vi "Set CCD_Config.vi"(8 "error in (no error)":errorcluster, 10 "input cluster":T1, 11 "Interface in":refnum<class "Interface.lvclass">) -> (0 "error out":errorcluster, 3 "Interface out":refnum<class "Interface.lvclass">)   [LabVIEW 2018, in "Interface.lvclass"]
uses:
  Interface.lvclass
  Interface.lvclass/Interface.ctl
panel:
  in  "EXPTIME":dbl
  in  "#FRAMES":u32
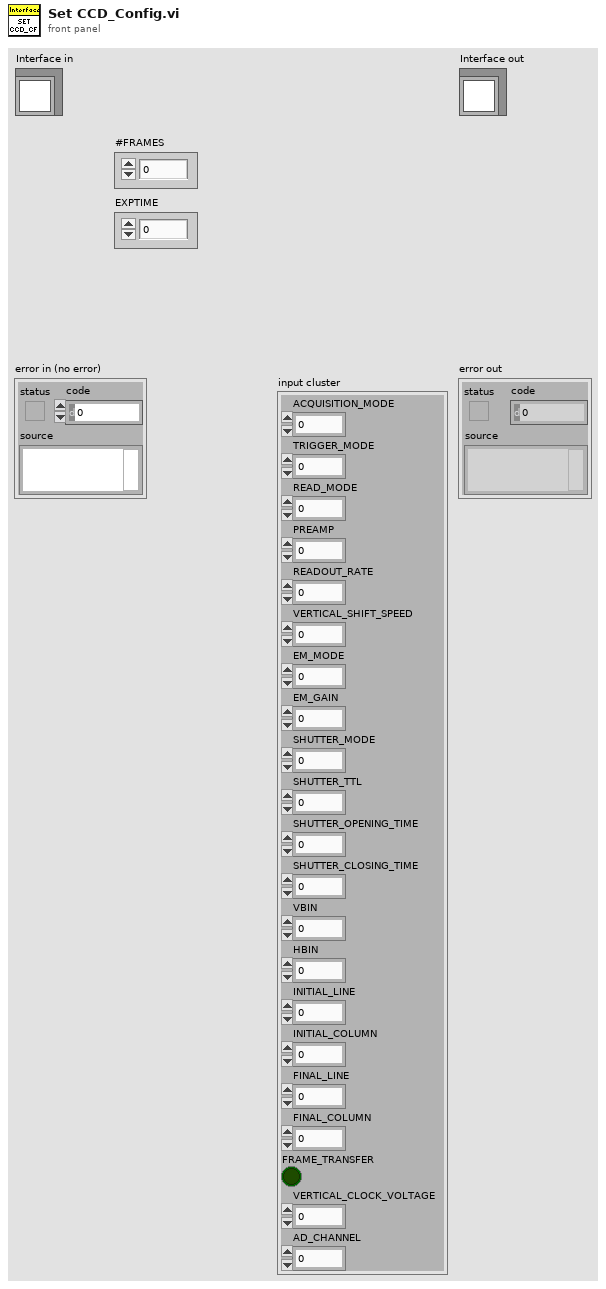
[diagram p1: front panel]
types:
  T1 = cluster{"ACQUISITION_MODE":u8, "TRIGGER_MODE":u8, "READ_MODE":u8, "PREAMP":u8, "READOUT_RATE":u8, "VERTICAL_SHIFT_SPEED":u8, "EM_MODE":u8, "EM_GAIN":u16, "SHUTTER_MODE":u8, "SHUTTER_TTL":u8, "SHUTTER_OPENING_TIME":u16, "SHUTTER_CLOSING_TIME":u16, "VBIN":u16, "HBIN":u16, "INITIAL_LINE":u16, "INITIAL_COLUMN":u16, "FINAL_LINE":u16, "FINAL_COLUMN":u16, "FRAME_TRANSFER":bool, "VERTICAL_CLOCK_VOLTAGE":u8, "AD_CHANNEL":u32}
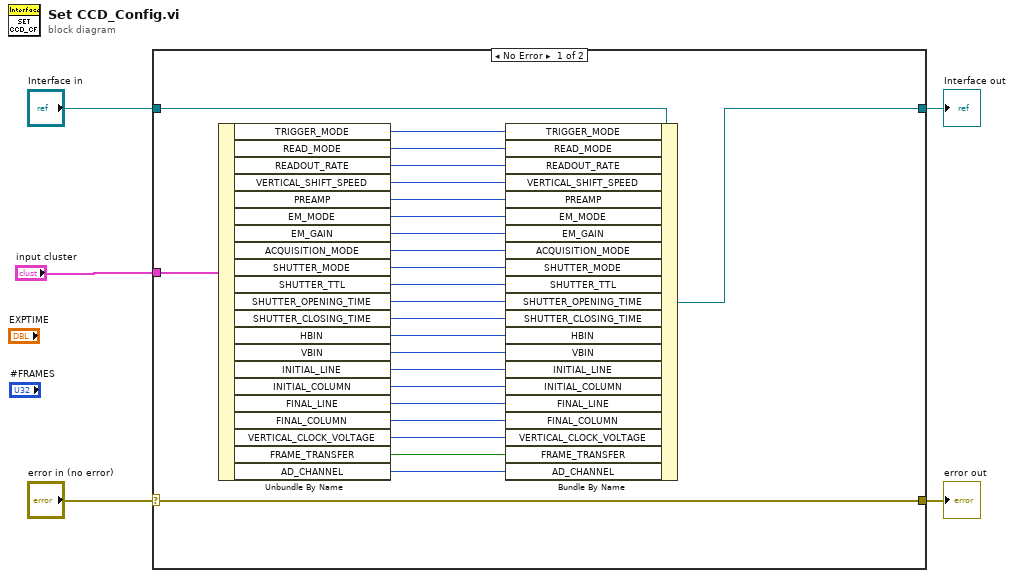
[diagram p0: block diagram]
diagram:
  n1 = case shown="No Error" "error in (no error)" {
    selector: "error in (no error)" -> [w30 w32]
    tunnel: [w30 w32] -> w4
    tunnel: [w6 w31] -> w2
    tunnel: "Interface in" -> [w7 w31]
    tunnel: "input cluster" -> [w8 _]
    frame No Error {
      n2 = Unbundle By Name(w8) -> ("TRIGGER_MODE"=w29:u8, "READ_MODE"=w28:u8, "READOUT_RATE"=w27:u8, "VERTICAL_SHIFT_SPEED"=w26:u8, "PREAMP"=w25:u8, "EM_MODE"=w24:u8, "EM_GAIN"=w23:u16, "ACQUISITION_MODE"=w22:u8, "SHUTTER_MODE"=w21:u8, "SHUTTER_TTL"=w20:u8, "SHUTTER_OPENING_TIME"=w19:u16, "SHUTTER_CLOSING_TIME"=w18:u16, "HBIN"=w17:u16, "VBIN"=w16:u16, "INITIAL_LINE"=w15:u16, "INITIAL_COLUMN"=w14:u16, "FINAL_LINE"=w13:u16, "FINAL_COLUMN"=w12:u16, "VERTICAL_CLOCK_VOLTAGE"=w11:u8, "FRAME_TRANSFER"=w10:bool, "AD_CHANNEL"=w9:u32)
      n3 = Bundle By Name(cluster=w7, "TRIGGER_MODE"=w29, "READ_MODE"=w28, "READOUT_RATE"=w27, "VERTICAL_SHIFT_SPEED"=w26, "PREAMP"=w25, "EM_MODE"=w24, "EM_GAIN"=w23, "ACQUISITION_MODE"=w22, "SHUTTER_MODE"=w21, "SHUTTER_TTL"=w20, "SHUTTER_OPENING_TIME"=w19, "SHUTTER_CLOSING_TIME"=w18, "HBIN"=w17, "VBIN"=w16, "INITIAL_LINE"=w15, "INITIAL_COLUMN"=w14, "FINAL_LINE"=w13, "FINAL_COLUMN"=w12, "VERTICAL_CLOCK_VOLTAGE"=w11, "FRAME_TRANSFER"=w10, "AD_CHANNEL"=w9) -> (w6:refnum<class "Interface.lvclass">)
    }
    frame Error {
    }
  }
  "error out" <- w4
  "Interface out" <- w2
